vi "Connect.vi"(8 "error in (no error)":errorcluster, 11 "Motion in":refnum<class "Motion.lvclass">) -> (0 "error out":errorcluster, 3 "Motion out":refnum<class "Motion.lvclass">)   [LabVIEW 2020, in "Motion.lvclass"]
uses:
  Motion.lvclass
  Motion.lvclass/Motion.ctl
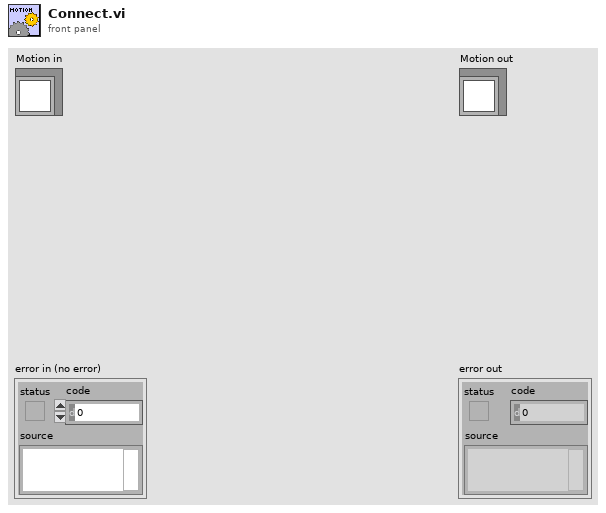
[diagram p1: front panel]
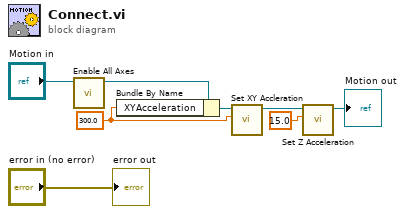
[diagram p0: block diagram]
diagram:
  w3 = 300.0 ("mm/s")
  n1 = call-dynamic "Enable All Axes.vi"("Motion in"="Motion in") -> ("Motion out"=w2:refnum<class "Motion.lvclass">)  [unwired: 9 in, 1 out]
  n2 = Bundle By Name(cluster=w2, "XYAcceleration"=w3) -> (w1:refnum<class "Motion.lvclass">)
  n3 = call-dynamic "Set XY Accleration.vi"("mm/s"=w3, "Motion in"=w1) -> ("Motion out"=w6:refnum<class "Motion.lvclass">)  [unwired: 8 in, 1 out]
  n4 = call-dynamic "Set Z Acceleration.vi"("mm/s"=15.0, "Motion in"=w6) -> ("Motion out"=→"Motion out":refnum<class "Motion.lvclass">)  [unwired: 8 in, 1 out]
  "error out" <- "error in (no error)"
